vi "Simulation Trace Element.vi"(8 "error in (no error)":errorcluster, 10 "Sensors Array":T1[](array[typedef]) {"accelerometer"."z axis (g)" format="%.3f"; "accelerometer"."y axis (g)" format="%.3f"; "accelerometer"."x axis (g)" format="%.3f"}, 11 "simulator":T7={"configuration"={"maxTime"=5.0, "enableVisualization"=TRUE, "Environment Definition"=path "simulation configuration.ini", "Record Location"=path "Simulation Record.xml", "autograde?"=TRUE, "interactive?"=FALSE, "Feedback Mode"=enum."debug navigation", "Robot State Charts"=[path "C:/Users/blueuser/Desktop/Robo Sim Berkley/cpsgrader-release-0.4/Simulators/EECS149lab/src/LabVIEW/statechart/Simulation Statechart.vi"], "statechart"=path "C:/Users/blueuser/Desktop/Robo Sim Berkley/cpsgrader-release-0.4/Simulators/EECS149lab/src/LabVIEW/statechart/Simulation Statechart.vi"}, "Statechart\ndisplay"=refnum, "first step?"=FALSE, "Robots Simulation Statecharts"=[], "Robots"=[]}) -> (0 "error out":errorcluster, 2 "trace element":T11 {"sensors"."accelerometer"."z axis (g)" format="%.3f"; "sensors"."accelerometer"."y axis (g)" format="%.3f"; "sensors"."accelerometer"."x axis (g)" format="%.3f"}, 3 "simulator":T7={"configuration"={"maxTime"=5.0, "enableVisualization"=TRUE, "Environment Definition"=path "simulation configuration.ini", "Record Location"=path "Simulation Record.xml", "autograde?"=TRUE, "interactive?"=FALSE, "Feedback Mode"=enum."debug navigation", "Robot State Charts"=[path "C:/Users/blueuser/Desktop/Robo Sim Berkley/cpsgrader-release-0.4/Simulators/EECS149lab/src/LabVIEW/statechart/Simulation Statechart.vi"], "statechart"=path "C:/Users/blueuser/Desktop/Robo Sim Berkley/cpsgrader-release-0.4/Simulators/EECS149lab/src/LabVIEW/statechart/Simulation Statechart.vi"}, "Statechart\ndisplay"=refnum, "first step?"=FALSE, "Robots Simulation Statecharts"=[], "Robots"=[]})   [LabVIEW 2014]
doc: "Reads parameters from the simulator sensors and packages them into a single trace element."
uses:
  Simulation Trace Element.ctl
  shared/Sensors.ctl
  shared/Accelerometer.ctl
  Kobuki/KobukiSensors.ctl
  Kobuki/Kobuki Bumps and WheelDrops.ctl
  Kobuki/Kobuki Buttons.ctl
  Kobuki/Charging Sources Available.ctl
  Simulated Position.ctl
  Simulated Orientation.ctl
  Simulator.ctl
  CyberSim interface/Simulation Configuration.ctl
  autograder/feedbackMode.ctl
  Multi Bot Code/RobotData.ctl
  <instrlib>/DC Motor Controller/HAIOL/DC Motor Controller.lvclass
  <vilib>/Robotics/Simulator/Interface/Simulator References/Get World Reference.vi
  <resource>/objmgr/LVODE.rc
  <vilib>/robotics/Simulator/NI_Robotics_Simulator.lvlib
  <vilib>/robotics/Kinematics/NI_Kinematics.lvlib
panel:
  # "Electrical: charging, battery, OI mode"
  # "Sensors: bump, cliff, button, wheel drop, wall, virtual wall"
  # "Motors:"
  # "Song"
  # "Inertia"
  # "Electrical: charging, battery, OI mode"
  # "Sensors: bump, cliff, button, wheel drop, wall, virtual wall"
  # "Motors:"
  # "Song"
  # "Inertia"
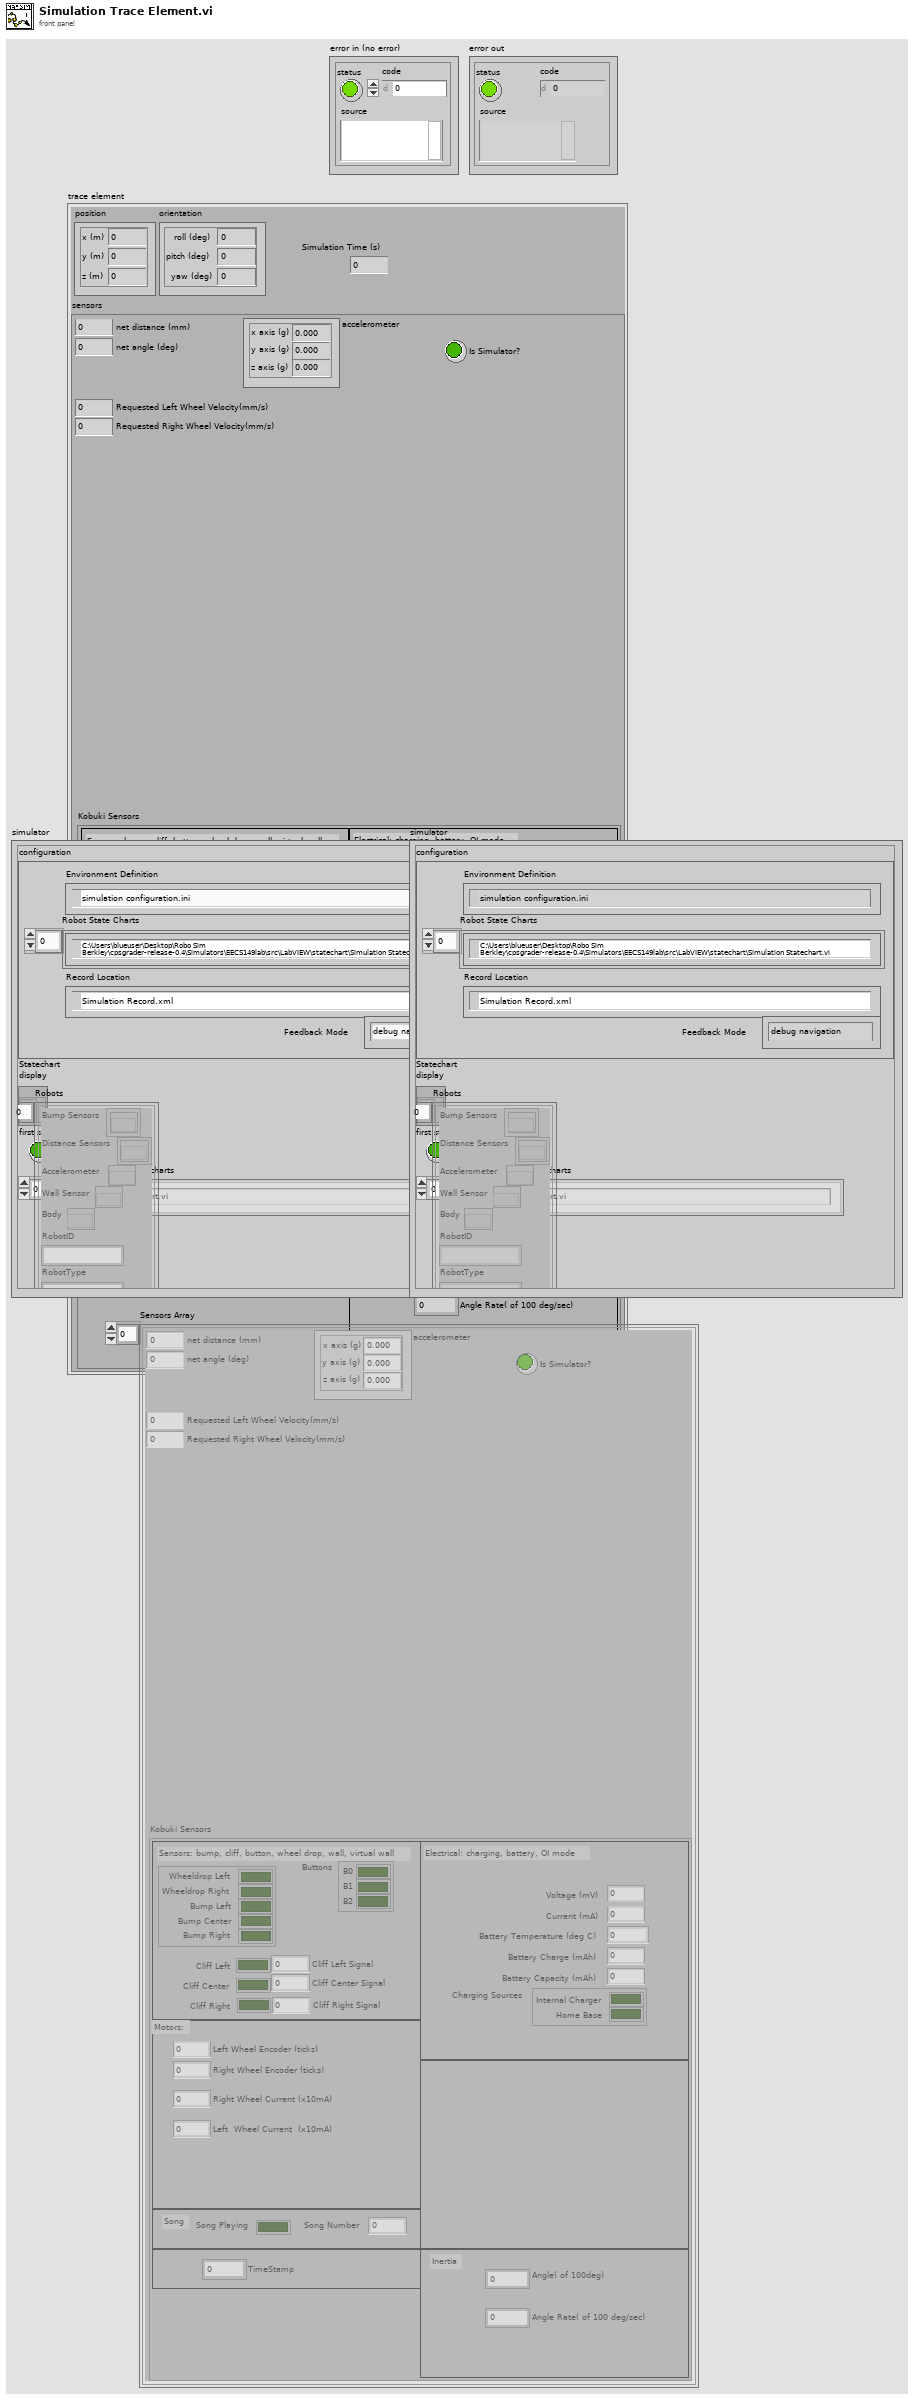
[diagram p1: front panel]
types:
  T1 = typedef "Sensors.ctl" = cluster{"net distance (mm)":i32, "net angle (deg)":i32, "accelerometer":T2, "Is Simulator?":bool, "Kobuki Sensors":T3, "Requested Left Wheel Velocity(mm/s)":i32, "Requested Right Wheel Velocity(mm/s)":i32}
  T2 = typedef "Accelerometer.ctl" = cluster{"x axis (g)":dbl, "y axis (g)":dbl, "z axis (g)":dbl}
  T3 = typedef "KobukiSensors.ctl" = cluster{"Bumps + Wheel Drops":T4, "Cliff Left":bool, "Cliff Center":bool, "Cliff Right":bool, "Cliff Left Signal":u16, "Cliff Center Signal":u16, "Cliff Right Signal":u16, "Buttons":T5, "Left Wheel Encoder (ticks)":u16, "Right Wheel Encoder (ticks) ":u16, "Right Wheel Current (x10mA)":i16, "Left  Wheel Current  (x10mA)":i16, "TimeStamp":u16, "Song Playing":bool, "Song Number":u8, "Voltage (mV)":i16, "Current (mA)":i16, "Battery Temperature (deg C)":i16, "Battery Charge (mAh)":i16, "Battery Capacity (mAh)":i16, "Charging Sources":T6, "Angle( of 100deg)":i16, "Angle Rate( of 100 deg/sec)":i16}
  T4 = typedef "Kobuki Bumps and WheelDrops.ctl" = cluster{"Wheeldrop Left":bool, "Wheeldrop Right":bool, "Bump Left":bool, "Bump Center":bool, "Bump Right":bool}
  T5 = typedef "Kobuki Buttons.ctl" = cluster{"B0":bool, "B1":bool, "B2":bool}
  T6 = typedef "Charging Sources Available.ctl" = cluster{"Internal Charger":bool, "Home Base":bool}
  T7 = typedef "Simulator.ctl" = cluster{"configuration":T8, "Statechart\ndisplay":refnum<vi>, "first step?":bool, "Robots Simulation Statecharts":path[], "Robots":T10[]}
  T8 = typedef "Simulation Configuration.ctl" = cluster{"maxTime":sgl, "enableVisualization":bool, "Environment Definition":path, "Record Location":path, "autograde?":bool, "interactive?":bool, "Feedback Mode":T9, "Robot State Charts":path[], "statechart":path}
  T9 = typedef "feedbackMode.ctl" = enum32{"debug navigation", "debug hill climb", "autograde navigation", "autograde hill climb"}
  T10 = typedef "RobotData.ctl" = cluster{"Bump Sensors":refnum<k20>[], "Distance Sensors":refnum<k20>[], "Accelerometer":refnum<k20>, "Wall Sensor":refnum<k20>, "Body":refnum<k20>, "RobotID":string, "RobotType":string, "Left Motor":refnum<class "DC Motor Controller.lvclass">, "Right Motor":refnum<class "DC Motor Controller.lvclass">}
  T11 = typedef "Simulation Trace Element.ctl" = cluster{"sensors":T1, "position":T12, "orientation":T13, "Simulation Time (s)":sgl}
  T12 = typedef "Simulated Position.ctl" = cluster{"x (m)":sgl, "y (m)":sgl, "z (m)":sgl}
  T13 = typedef "Simulated Orientation.ctl" = cluster{"roll (deg)":sgl, "pitch (deg)":sgl, "yaw (deg)":sgl}
  T14 = cluster{"Position[0]":sgl, "Position[1]":sgl, "Position[2]":sgl}
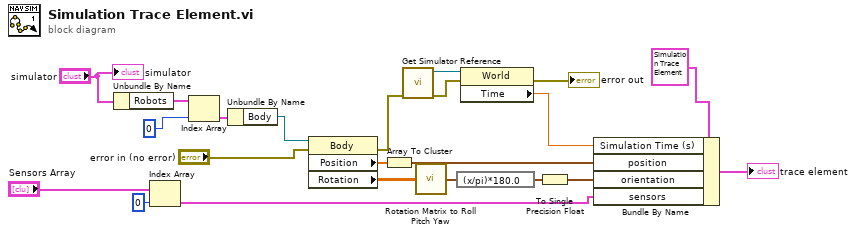
[diagram p0: block diagram]
diagram:
  n1 = Unbundle By Name("simulator") -> ("Robots"=w9:T10[])
  n2 = Index Array(array="Sensors Array", index=0) -> (element=w1:T1)
  n3 = Index Array(array=w9, index=0) -> (element=w8:T10)
  n4 = Unbundle By Name(w8) -> ("Body"=w7:refnum<k20>)
  n5 = property class="Body"(reference=w7, error in="error in (no error)") -> (error out=w20:errorcluster, "Position"=w16:sgl[], "Rotation"=w11:sgl[][])  [unwired: 1 out]
  n6 = Array To Cluster(array=w16) -> (cluster=w15:T14)
  n7 = call-poly <vilib>:"Get Simulator Reference.vi"("error in (no error)"=w20) -> ("error out"=w21:errorcluster, "world ref"=w22:refnum<k20>)  [unwired: 9 in]
  n8 = call <vilib>:"Rotation Matrix to Roll Pitch Yaw.vi"("rotation matrix"=w11) -> ("angles"=w14:cluster{"roll":dbl, "pitch":dbl, "yaw":dbl})
  n9 = expression code="(x/pi)*180.0" ("radians to degrees")(w14) -> (w13:cluster{"roll":dbl, "pitch":dbl, "yaw":dbl})
  n10 = property class="World"(reference=w22, error in=w21) -> (error out=→"error out":errorcluster, "Time"=w17:sgl)  [unwired: 1 out]
  n11 = To Single Precision Float(number=w13) -> (single precision float=w12:cluster{"roll":sgl, "pitch":sgl, "yaw":sgl})
  n12 = Bundle By Name(cluster=T11 {"sensors"={"net distance (mm)"=0, "net angle (deg)"=0, "accelerometer"={"x axis (g)"=0.0, "y axis (g)"=0.0, "z axis (g)"=0.0}, "Is Simulator?"=FALSE, "Kobuki Sensors"={"Bumps + Wheel Drops"={"Wheeldrop Left"=FALSE, "Wheeldrop Right"=FALSE, "Bump Left"=FALSE, "Bump Center"=FALSE, "Bump Right"=FALSE}, "Cliff Left"=FALSE, "Cliff Center"=FALSE, "Cliff Right"=FALSE, "Cliff Left Signal"=0, "Cliff Center Signal"=0, "Cliff Right Signal"=0, "Buttons"={"B0"=FALSE, "B1"=FALSE, "B2"=FALSE}, "Left Wheel Encoder (ticks)"=0, "Right Wheel Encoder (ticks) "=0, "Right Wheel Current (x10mA)"=0, "Left  Wheel Current  (x10mA)"=0, "TimeStamp"=0, "Song Playing"=FALSE, "Song Number"=0, "Voltage (mV)"=0, "Current (mA)"=0, "Battery Temperature (deg C)"=0, "Battery Charge (mAh)"=0, "Battery Capacity (mAh)"=0, "Charging Sources"={"Internal Charger"=FALSE, "Home Base"=FALSE}, "Angle( of 100deg)"=0, "Angle Rate( of 100 deg/sec)"=0}, "Requested Left Wheel Velocity(mm/s)"=0, "Requested Right Wheel Velocity(mm/s)"=0}, "position"={"x (m)"=0.0, "y (m)"=0.0, "z (m)"=0.0}, "orientation"={"roll (deg)"=0.0, "pitch (deg)"=0.0, "yaw (deg)"=0.0}, "Simulation Time (s)"=0.0} ("trace element"), "Simulation Time (s)"=w17, "position"=w15, "orientation"=w12, "sensors"=w1) -> (→"trace element":T11)
  "simulator" <- "simulator"
